vi "FTW-CodeGen-Prototype.vi"(0 "ADAPT_Type and Defaults":cluster{"Element":variant}, 5 "REPLACE_JSON String":string, 7 "REPLACE_Element Path":string, 11 "REPLACE_error in":errorcluster) -> (4 "ADAPT_Values":cluster{"Element":variant}, 15 "REPLACE_error out":errorcluster)   [LabVIEW 2014, in "FTW-JSON-Deserialize.xnode"]
uses:
  FTW-JSON-Deserialize.xnode
  error/FTW-ERR-NoErrorConstant.vi
  error/FTW-ERR-ThrowError.vi
  error/FTW-ERR-CallChain.vi
  string/FTW-STR-ReplaceWhitespace.vi
panel:
  # "Inputs"
  # "Outputs"
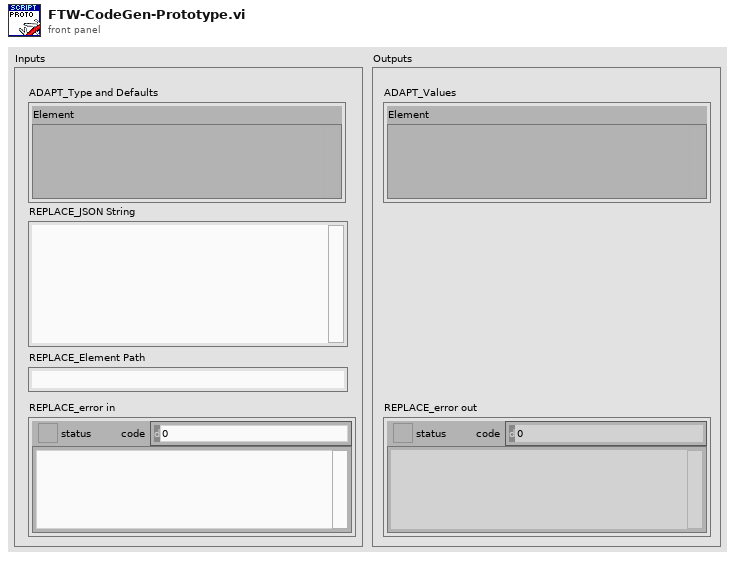
[diagram p1: front panel]
types:
  T1 = typedef "FTW-Reflection-Types.ctl" = enum16{"Unknown", "Void", "Array", "Cluster", "LVObject", "Boolean", "I8", "I16", "I32", "I64", "U8", "U16", "U32", "U64", "SGL", "DBL", "EXT", "CSG", "CDB", "CXT", "FXP", "EnumU8", "EnumU16", "EnumU32", "EnumU64", "SGLwithUnit", "DBLwithUnit", "EXTwithUnit", "CSGwithUnit", "CDBwithUnit", "CXTwithUnit", "String", "Path", "Picture", "Tag", "LVVariant", "Timestamp", "WaveformI8", "WaveformI16", "WaveformI32", "WaveformI64", "WaveformU8", "WaveformU16", "WaveformU32", "WaveformU64", "WaveformSGL", "WaveformDBL", "WaveformEXT", "WaveformCSG", "WaveformCDB", "WaveformCXT", "WaveformDigital", "WaveformUnknownType", "DigitalData", "DynamicData", "ExternalData", "FileByteStream", "TDMStream", "dotNET", "ActiveX", "VIServerReference", "VIReference", "ApplicationInstance", "Menu", "ConnectionDataSocket", "ConnectionVISA", "ConnectionBluetooth", "ConnectionIrDA", "ConnectionTCP", "ConnectionUDP", "ConnectionHTTPClient", "ConnectionFTP", "Occurrence", "Notifier", "Queue", "Rendezvous", "Semaphore", "RTFIFO", "EventPublisher", "EventRegistration", "EventCallback", "DataValueReference", "GenericClass", "GenericClassTag", "GenericClassDeepCopy", "GenericClassFlattened", "GenericClassTagFlattened", "GenericReferenceType", "WindowsRegistry", "OverloadedDatalogRef", "ReferenceUnknownType"}
  T2 = typedef "FTW-JSON-Type.ctl" = enum16{"Object", "Array", "String", "Integer", "Floating Point", "true", "false", "null", "undefined"}
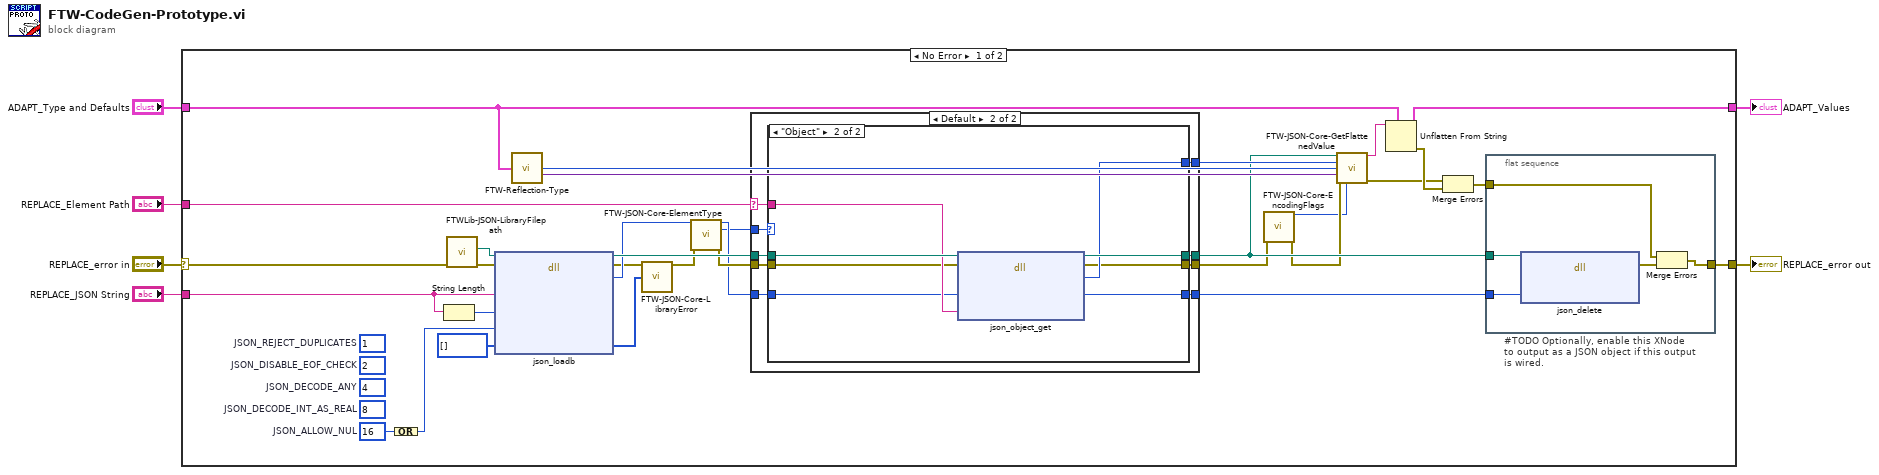
[diagram p0: block diagram]
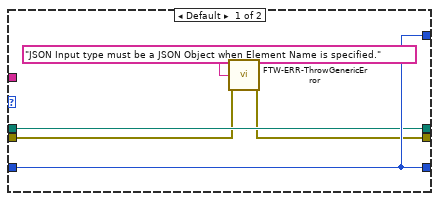
[diagram p3: hidden frame]
diagram:
  n1 = case shown="No Error" "REPLACE_error in" {
    selector: "REPLACE_error in" -> [w31 w70]
    tunnel: "REPLACE_JSON String" -> [w30 _]
    tunnel: [w29 w70] -> w2
    tunnel: "ADAPT_Type and Defaults" -> [w38 w69]
    tunnel: [w37 w69] -> w4
    tunnel: "REPLACE_Element Path" -> [w13 _]
    frame No Error {
      w32 = u64 16  # JSON_ALLOW_NUL
      (unwired) u64 8  # JSON_DECODE_INT_AS_REAL
      (unwired) u64 4  # JSON_DECODE_ANY
      (unwired) u64 2  # JSON_DISABLE_EOF_CHECK
      (unwired) u64 1  # JSON_REJECT_DUPLICATES
      n2 = Compound Arithmetic op=OR(w32) -> (w33:u64)
      n3 = String Length(string=w30) -> (length=w34:i32)
      n4 = call "FTWLib-JSON-LibraryFilepath.vi"("error in"=w31) -> ("error out"=w36:errorcluster, "JSON Library Filepath"=w35:path)  [unwired: 9 in]
      n5 = dll-call lib="?" fn="json_loadb"(path in=w35, error in=w36, "JSON Buffer"=w30, "Buffer Size"=w34, "Flags"=w33, "Error Structure"=u8[] []) -> (path out=w25:path, error out=w20:errorcluster, "JSON Object Pointer"=w22:i64, "Error Structure"=w18:u8[])  [unwired: 4 in]
      n6 = call "FTW-Reflection-Type.vi"("Anything"=w38) -> ("LabVIEW Type"=w27:T1, "Variant Type and Value"=w26:variant)  [unwired: 12 in, 1 out]
      n7 = call "FTW-JSON-Core-LibraryError.vi"("error in"=w20, "Error Structure"=w18) -> ("error out"=w19:errorcluster)  [unwired: 13 in]
      n8 = call "FTW-JSON-Core-ElementType.vi"("JSON Element"=w22, "error in"=w19) -> ("JSON Element out"=w21:i64, "JSON Type"=w14:T2, "error out"=w23:errorcluster)  [unwired: 11 in]
      n9 = case shown="Default" w13 {
        selector: w13 -> [_ w47]
        tunnel: w25 -> [w45 w55]
        tunnel: [w45 w54] -> w10
        tunnel: [w46 w53] -> w24
        tunnel: w23 -> [w44 w52]
        tunnel: w21 -> [w46 w51]
        tunnel: [w46 w50] -> w11
        tunnel: [w44 w49] -> w8
        tunnel: w14 -> [_ w48]
        frame "" {
        }
        frame Default {
          n10 = case shown="\"Object\"" w48 {
            tunnel: w55 -> [w58 w68]
            tunnel: [w58 w67] -> w54
            tunnel: [w59 w66] -> w53
            tunnel: w47 -> [_ w65]
            tunnel: w52 -> [w57 w64]
            tunnel: w51 -> [w59 w63]
            tunnel: [w59 w62] -> w50
            tunnel: [w56 w61] -> w49
            frame Default {
              n11 = call "FTW-ERR-ThrowGenericError.vi"("Error Message"="JSON Input type must be a JSON Object when Element Name is specified.", "error in"=w57) -> ("error out"=w56:errorcluster)  [unwired: 13 in]
            }
            frame "Object" {
              n12 = dll-call lib="?" fn="json_object_get"(path in=w68, error in=w64, "JSON Object Pointer"=w63, "Element Key"=w65) -> (path out=w67:path, error out=w61:errorcluster, "JSON Element Pointer"=w62:i64, "JSON Object Pointer"=w66:i64)  [unwired: 2 in]
            }
          }
        }
      }
      n13 = call "FTW-JSON-Core-EncodingFlags.vi"("error in"=w8) -> ("Encoding Flags"=w7:i64, "error out"=w9:errorcluster)  [unwired: 13 in]
      n14 = call "FTW-JSON-Core-GetFlattenedValue.vi"("JSON Library Filepath"=w10, "JSON Element"=w11, "LabVIEW Type"=w27, "Element Default Value"=w26, "error in"=w9, "Encoding Flags"=w7) -> ("Flattened Value"=w17:string, "error out"=w15:errorcluster)  [unwired: 8 in]
      n15 = Unflatten From String(type=w38, binary string=w17) -> (value=w37:cluster{"Element":variant}, error out=w16:errorcluster)  [unwired: 3 in, 1 out]
      n16 = Merge Errors(w15, w16) -> (w28:errorcluster)
      n17 = flat-sequence "#TODO Optionally, enable this XNode\nto output as a JSON object if this output\nis wired." {
        tunnel: [w43] -> w29
        tunnel: w28 -> [w42]
        tunnel: w24 -> [w41]
        tunnel: w10 -> [w39]
        frame #0 {
          n18 = dll-call lib="?" fn="json_delete"(path in=w39, "JSON Object Pointer"=w41) -> (error out=w40:errorcluster)  [unwired: 4 in, 1 out]
          n19 = Merge Errors(w42, w40) -> (w43:errorcluster)
        }
      }
    }
    frame Error {
    }
  }
  "REPLACE_error out" <- w2
  "ADAPT_Values" <- w4
